vi "Convert Scanned HEX data to ASCII QR Code.vi"(11 "Scanned HEX data":string) -> (3 "ASCII QR Code":string)   [LabVIEW 2023]
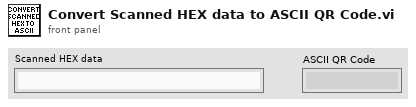
[diagram p1: front panel]
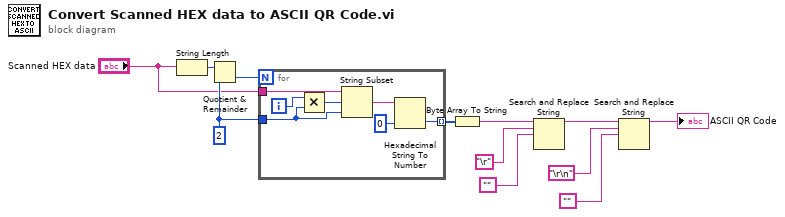
[diagram p0: block diagram]
diagram:
  w9 = 2 ("y")
  n1 = String Length(string="Scanned HEX data") -> (length=w11:i32)
  n2 = Quotient & Remainder(x=w11, y=w9) -> (floor(x/y)=w10:i32)  [unwired: 1 out]
  n3 = for {
    N: w10 -> [_]
    tunnel: "Scanned HEX data" -> [w17]
    tunnel: [w18] -> w12 mode=indexing
    tunnel: w9 -> [w13]
    i -> [w14]
    n4 = Multiply(x=w14, y=w13) -> (x*y=w15:i32)
    n5 = String Subset(string=w17, offset (0)=w15, length (rest)=w13) -> (substring=w16:string)
    n6 = Hexadecimal String To Number(string=w16, default (0uL)=u8 0) -> (number=w18:u8)  [unwired: 1 in, 1 out]
  }
  n7 = Byte Array To String(unsigned byte array=w12) -> (string=w7:string)
  n8 = Search and Replace String(input string=w7, search string="\r", replace string="") -> (result string=w6:string)  [unwired: 5 in, 3 out]
  n9 = Search and Replace String(input string=w6, search string="\r\n", replace string="") -> (result string=→"ASCII QR Code":string)  [unwired: 5 in, 3 out]
